vi "_Strip apostrophe - array.vi"(11 "string":string[](array[string])) -> (3 "content":string[](array[string]))   [LabVIEW 2014, in "_lvcicd_support_2014.lvlib"]
uses:
  _lvcicd_support_2014.lvlib
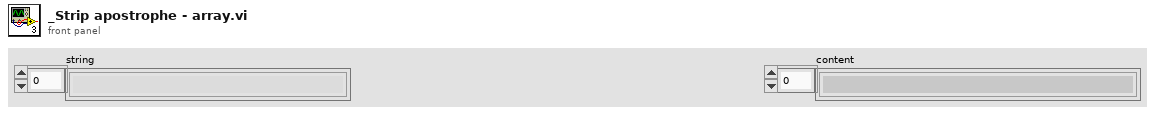
[diagram p1: front panel]
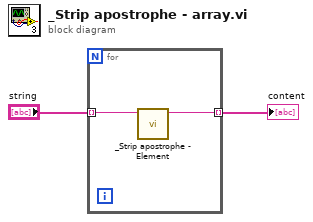
[diagram p0: block diagram]
diagram:
  n1 = for {
    tunnel: "string" -> [w4] mode=indexing
    tunnel: [w3] -> w1 mode=indexing
    n2 = call "_Strip apostrophe - Element.vi"("string"=w4) -> ("s? t:f"=w3:string)  [unwired: 10 in]
  }
  "content" <- w1
